vi "Register gRPC Server.vi"(8 "error in (no error)":errorcluster, 10 "gRPC ID":T1, 11 "CIFTemplatePlugin in":refnum<class "Template_Plugin.lvclass">) -> (0 "error out":errorcluster, 2 "gRPC ID Out":T1, 3 "CIFTemplatePlugin out":refnum<class "Template_Plugin.lvclass">)   [LabVIEW 2021, in "Template_Plugin.lvclass"]
uses:
  Template_Plugin.lvclass
  Template_Plugin.lvclass/Template_Plugin.ctl
  <vilib>/CIF Foundation/CIF Core/CIFCore/Class/CIFCorePlugin.lvclass
  Grpc/Template_server/Template_server.lvlib
  Grpc/Template_server/RPC Service/Template/Template.lvclass
  C:/Program Files/National Instruments/LabVIEW 2021/vi.lib/gRPC/LabVIEW gRPC Servicer/ServiceBase/ServiceBase.lvclass
  D:/dev/Plugins/Template/src/Template/Grpc/Template_server/RPC Service/Template/Template.lvclass
  C:/Program Files/National Instruments/LabVIEW 2021/vi.lib/CIF Foundation/CIF Core/CIFCore/Class/CIFCorePlugin.lvclass
  D:/dev/Plugins/Template/src/Template/Class/Template_Plugin.lvclass
  <vilib>/gRPC/LabVIEW gRPC Library/Shared/grpcId.ctl
  <vilib>/gRPC/LabVIEW gRPC Library/grpc-lvsupport-release.lvlib
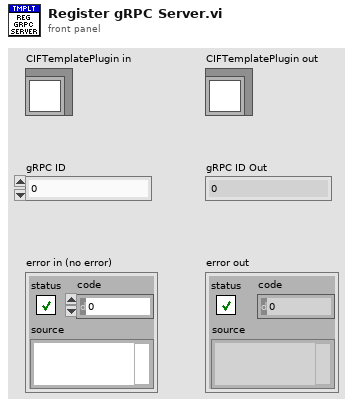
[diagram p1: front panel]
types:
  T1 = typedef "grpc-lvsupport-release.lvlib/grpcId.ctl" = u64
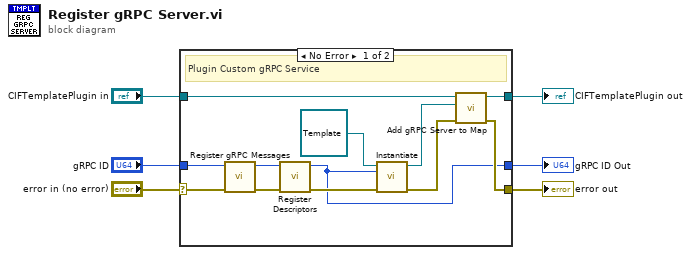
[diagram p0: block diagram]
diagram:
  n1 = case shown="No Error" "error in (no error)" {
    selector: "error in (no error)" -> [w7 w21]
    tunnel: [w13 w21] -> w1
    tunnel: [w17 w20] -> w3
    tunnel: "CIFTemplatePlugin in" -> [w18 w20]
    tunnel: "gRPC ID" -> [w8 w19]
    tunnel: [w9 w19] -> w2
    frame No Error {
      # "Plugin Custom gRPC Service"
      n2 = call "Register gRPC Messages.vi"("error in (no error)"=w7, "gRPC ID"=w8) -> ("error out"=w12:errorcluster, "gRPC ID Out"=w11:T1)  [unwired: 8 in]
      n3 = call "Register Descriptors.vi"("error in (no error)"=w12, "gRPC ID"=w11) -> ("error out"=w10:errorcluster, "gRPC ID Out"=w9:T1)  [unwired: 8 in]
      n4 = call-dynamic "Instantiate.vi"("error in"=w10, "gRPCid"=w9, "iService"=refnum<class "Template.lvclass"> refnum ("CIF_Plugin_Core_server.lvlib:PluginCore.lvclass")) -> ("error out"=w15:errorcluster, "iService"=w14:refnum<class "Template.lvclass">)  [unwired: 7 in]
      n5 = call <vilib>:"Add gRPC Server to Map.vi"("error in (no error)"=w15, "gRPC Server Class"=w14, "CIFTemplateNode in"=w18) -> ("error out"=w13:errorcluster, "CIFTemplateNode in"=w17:refnum<class "Template_Plugin.lvclass">)  [unwired: 7 in]
    }
    frame Error {
    }
  }
  "error out" <- w1
  "CIFTemplatePlugin out" <- w3
  "gRPC ID Out" <- w2
